vi "ScanningWaveform_v5.vi"(0 "Vy-min":dbl, 1 "Vy-max":dbl, 2 "yPixels/tPixels":dbl, 3 "xPixels/rPixels":dbl, 4 "Vx-min":dbl, 5 "Vx-max":dbl, 6 "Drawing Mode":u16(ring) items=["Image", "Fill Rectangle", "Fill Circle", "Draw Freeform", "Fill Freeform", "Ellipse Boundary", "Line"], 7 "Angle":dbl, 8 "Scanning Mode":u16(ring) items=["Raster", "Spiral"], 9 "AOrate":dbl, 10 "Points":cluster{"X":dbl, "Y":dbl}[](array[cluster]), 11 "points in ellipse":dbl) -> (12 "numPixels":dbl, 13 "Y-WaveArray":dbl[](array[numeric]), 14 "P":dbl, 19 "X-WaveArray":dbl[](array[numeric]))   [LabVIEW 2015]
panel:
  out "Y Graph 2":dbl[](graph)
  out "min":dbl
  out "max":dbl
  out "flyback time (us)":dbl
  out "C":dbl
  out "Sx":dbl
  out "S":dbl
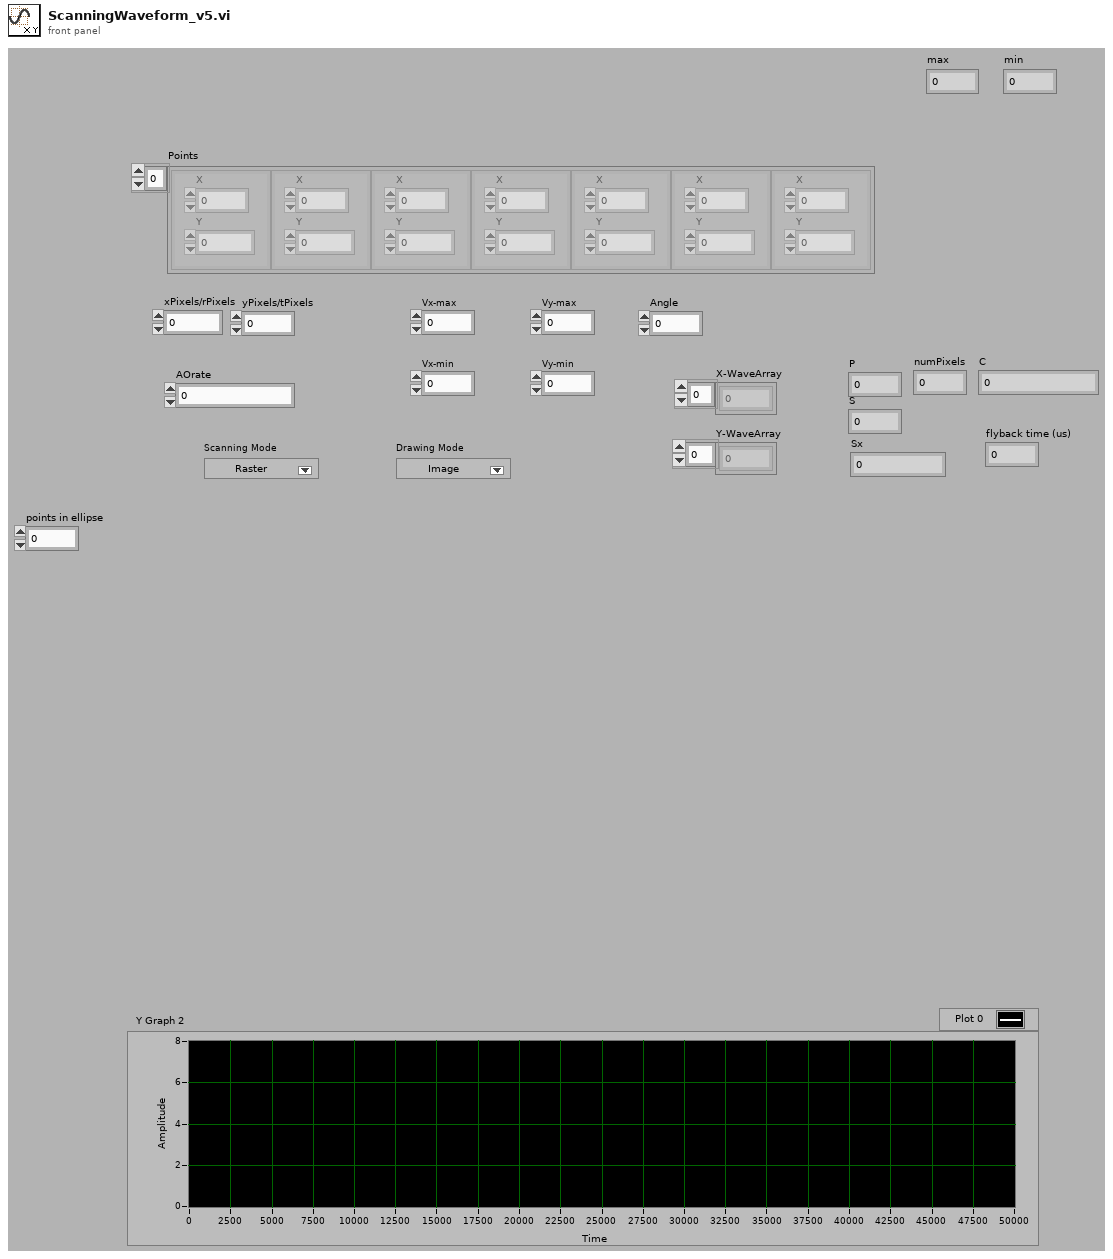
[diagram p1: front panel]
types:
  T1 = typedef "LVRectTypeDef.ctl" = cluster{"Left":i16, "Top":i16, "Right":i16, "Bottom":i16}
  T2 = cluster{"Xpixels":i32, "Vxminref":dbl, "Vxmaxref":dbl, "P":dbl, "Ypixels":i32, "Vyminref":dbl, "Vymaxref":dbl, "srate":sgl, "sAOxy":i32, "timeout":dbl, "type":string, "date":string, "time":string, "Colormap":u16, "Drawing Mode":u16, "Scanning Mode":u16, "square pixels":bool, "square matrix":bool, "Xpixels Img":i32, "Vx-min Img":dbl, "VX-max Img":dbl, "Ypixels Img":i32, "Vy-min Img":dbl, "Vy-max Img ":dbl, "Angle Img":dbl, "autoshutter":bool, "finite":bool, "cont":bool, "wavdet":bool, "measpoints":i32, "avpp":i32, "bufferAO":i32, "bufferAI":i32, "starttick":u32, "waveform":path, "Vx-ref":dbl, "Vy-ref":dbl, "refreshrate":dbl, "refreshbuffer":i32, "tt_cycles":i32, "motorref":refnum<k7>, "mirrorswitch":refnum<k7>, "sample mode":i32, "maxbufferAI":i32, "srateAODO":sgl, "bin":sgl, "Pel":sgl, "Angle draw":dbl, "srate Img":sgl, "ROIimg_plotbounds":T1, "auto OD":bool, "ODfilt":u16, "aAI":i32[], "aCI":i32[], "aAO":u32[], "aDO":u32[], "refwfsize":dbl, "Lifetime":bool, "Vz-Img":dbl, "Vz-ref":dbl, "Vz-reset":dbl, "AIoverride":bool, "aAS":u32[], "XYZstart":dbl[]}
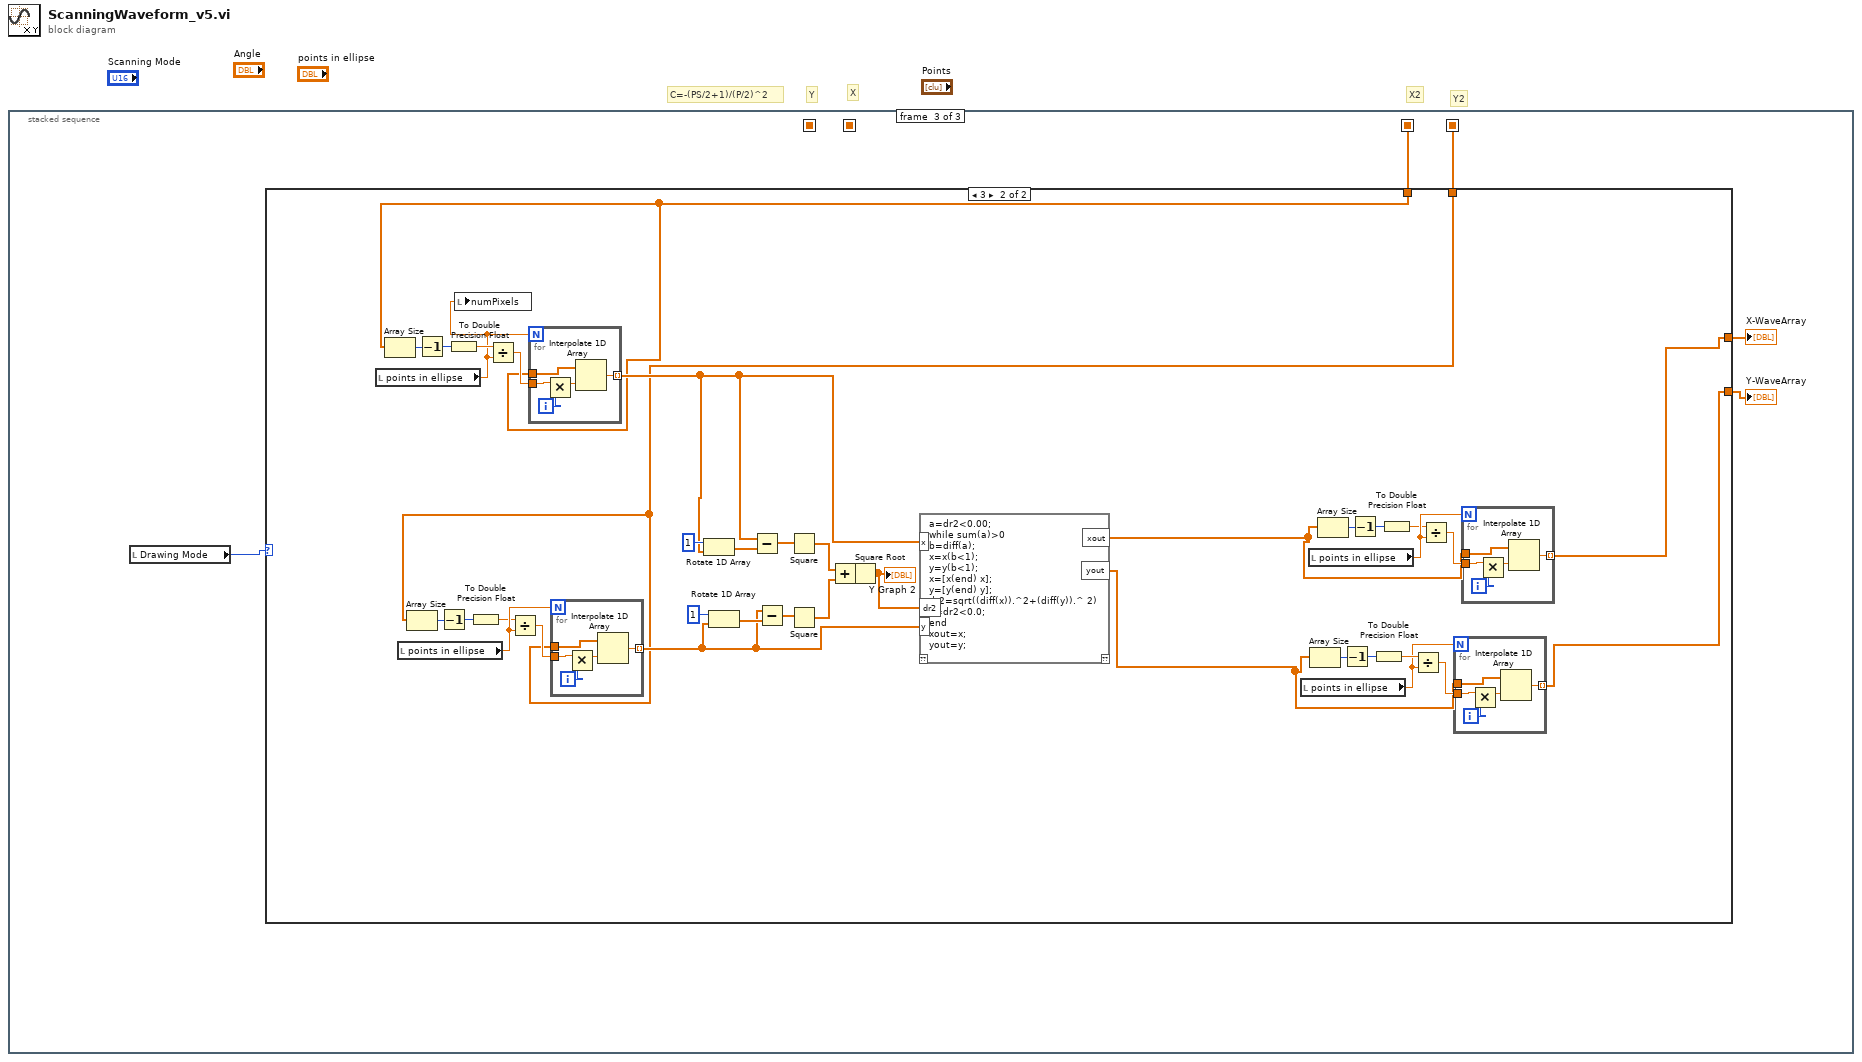
[diagram p0: block diagram]
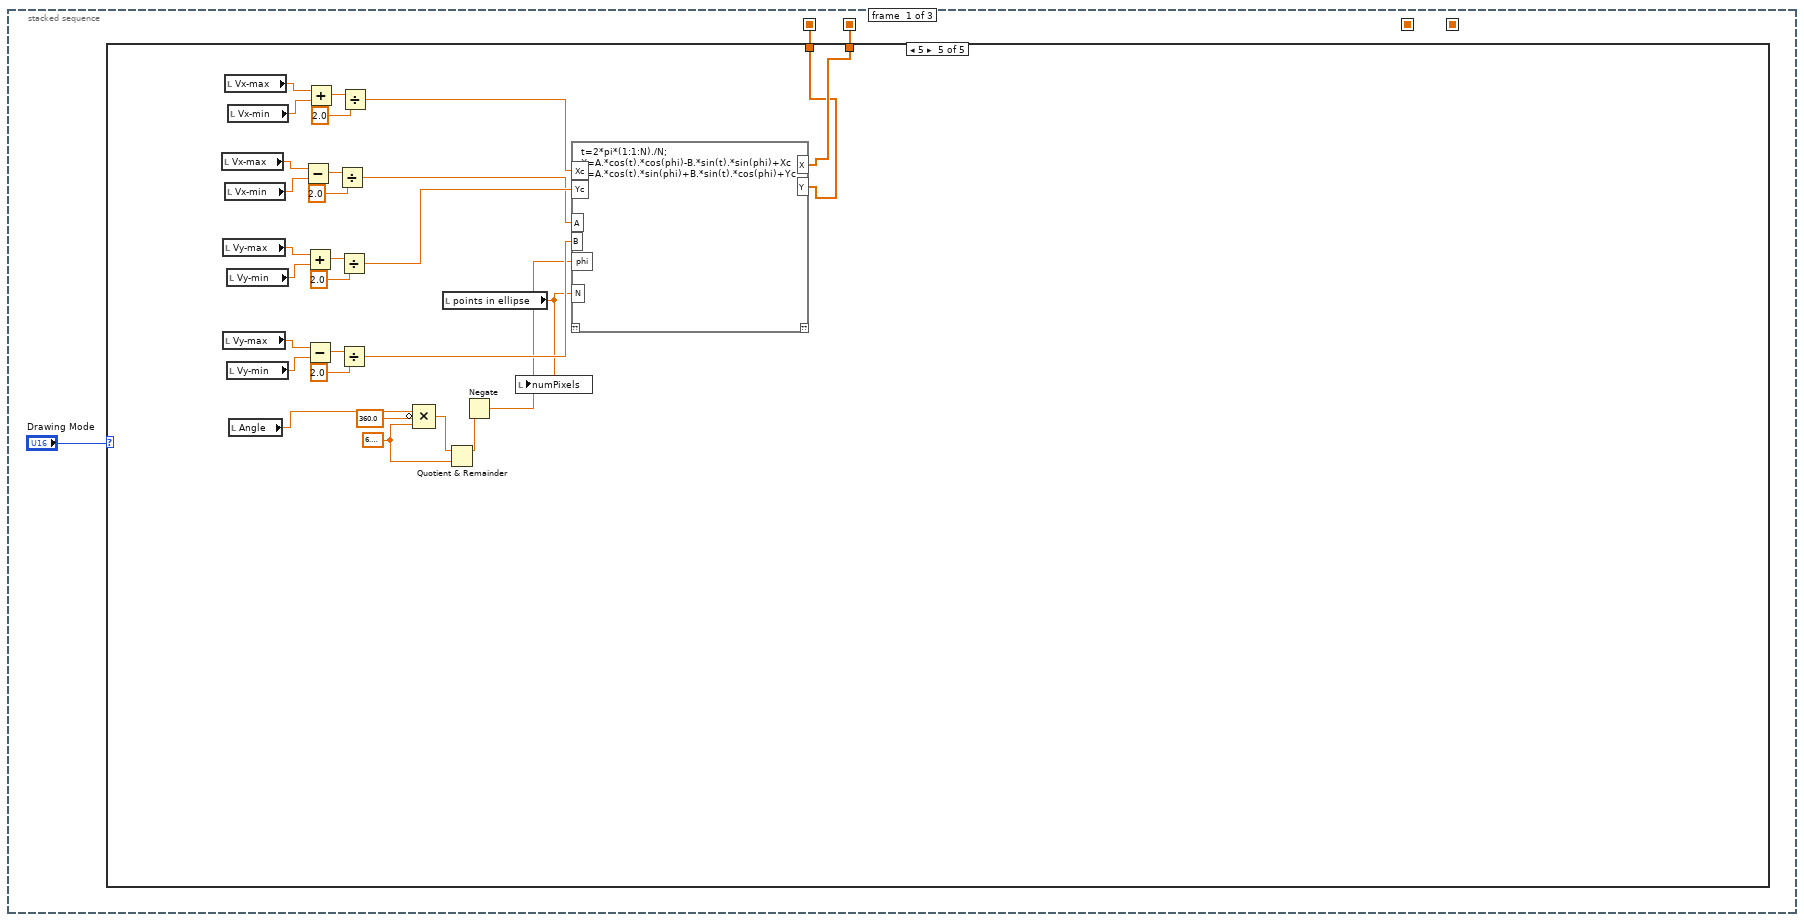
[diagram p2: hidden frame]
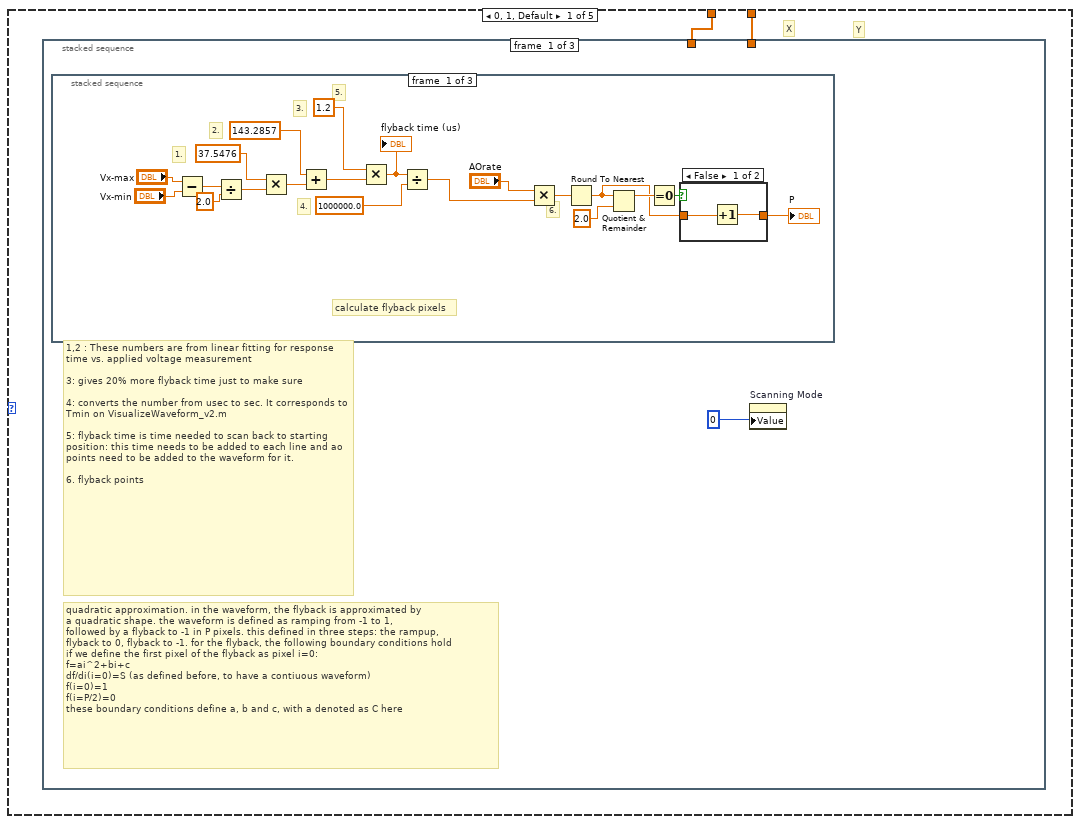
[diagram p3: hidden frame]
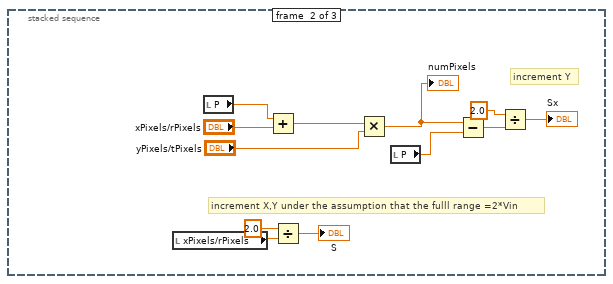
[diagram p5: hidden frame]
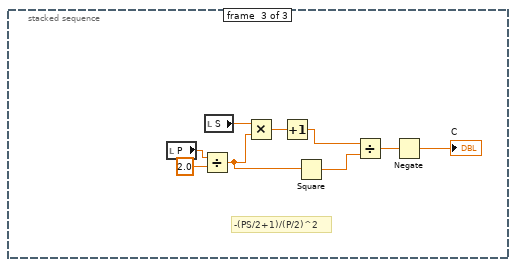
[diagram p6: hidden frame]
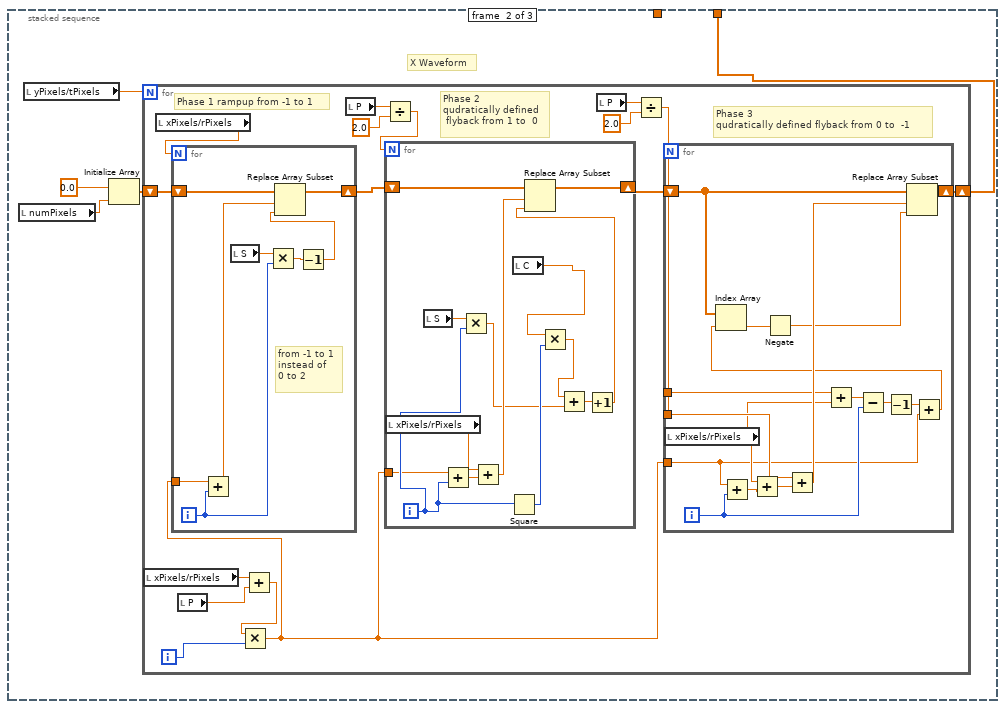
[diagram p7: hidden frame]
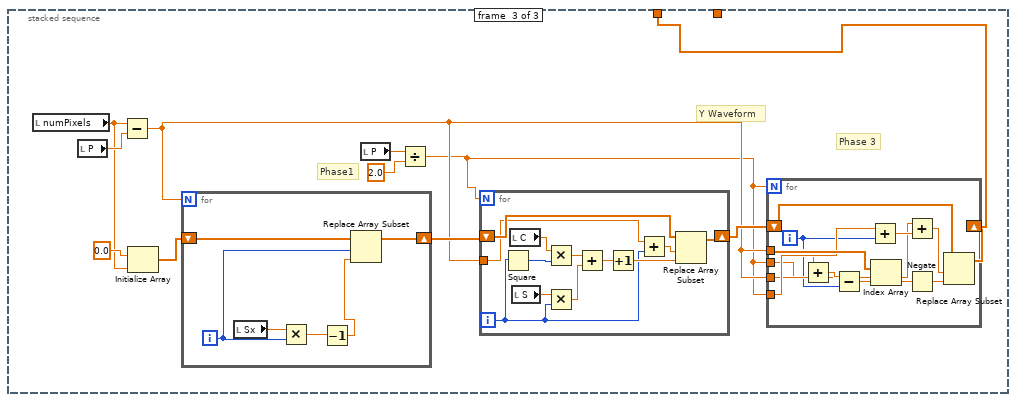
[diagram p8: hidden frame]
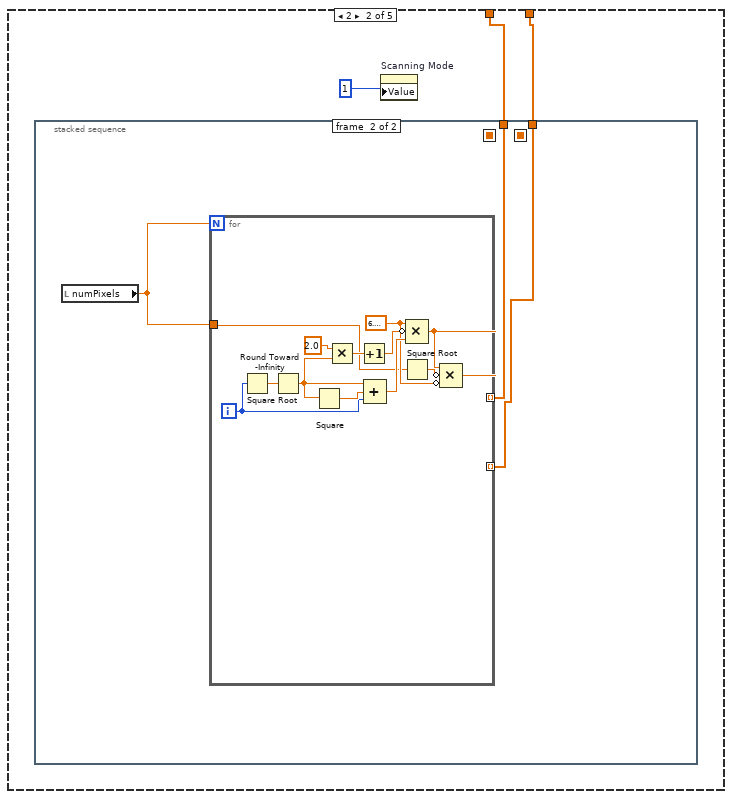
[diagram p9: hidden frame]
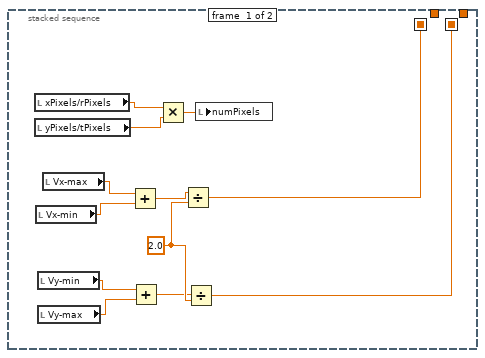
[diagram p10: hidden frame]
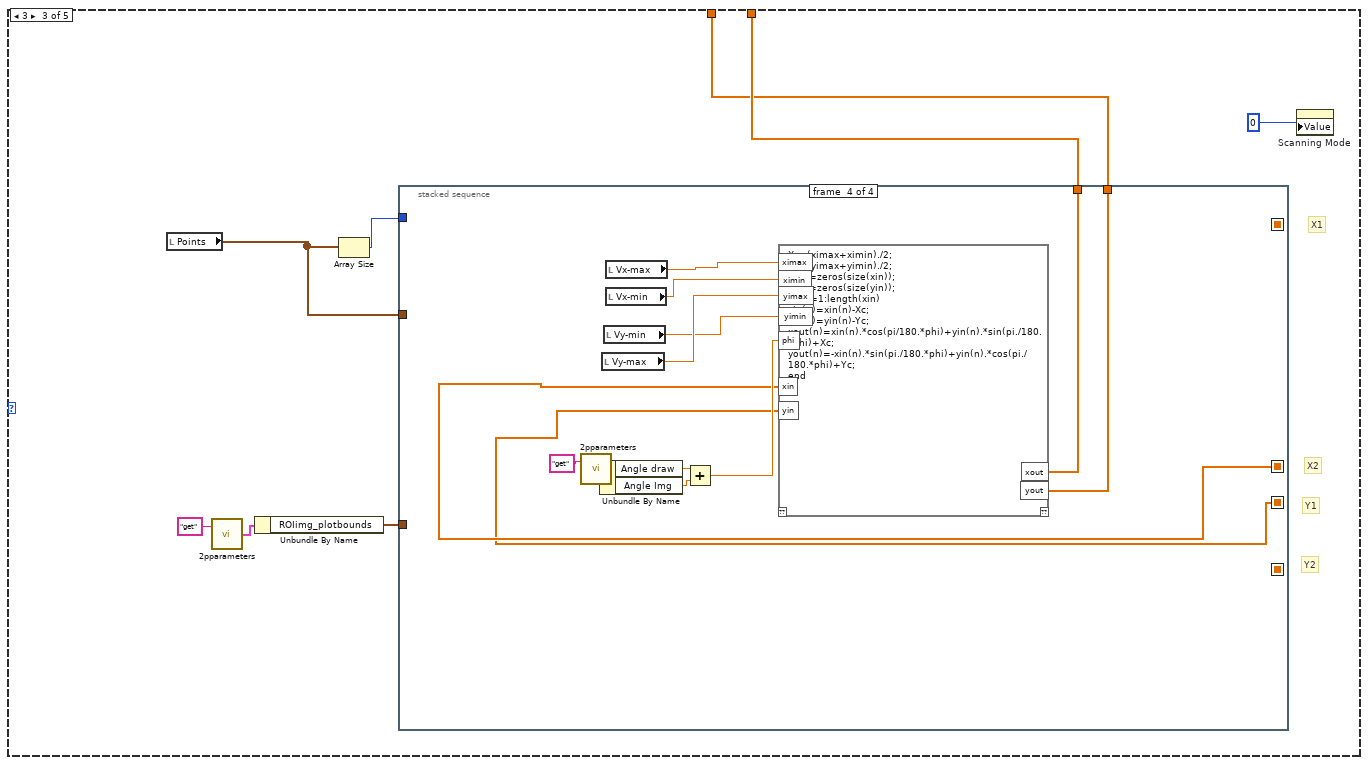
[diagram p11: hidden frame]
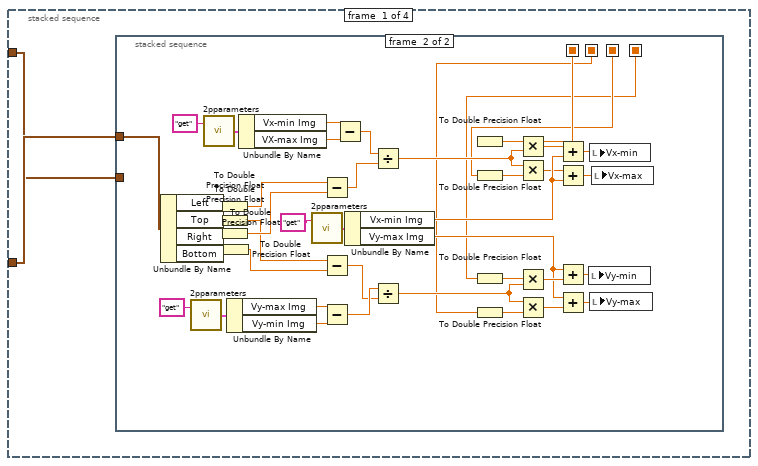
[diagram p12: hidden frame]
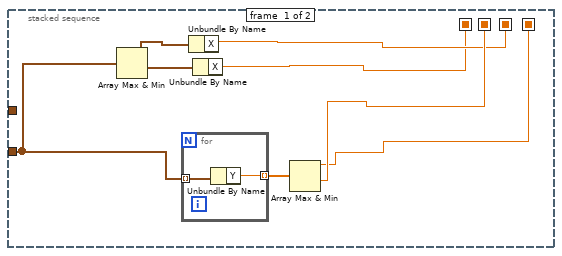
[diagram p13: hidden frame]
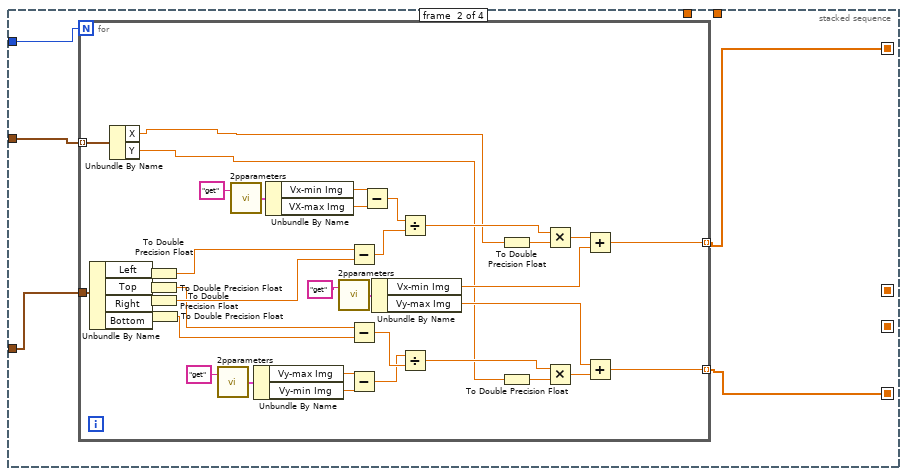
[diagram p14: hidden frame]
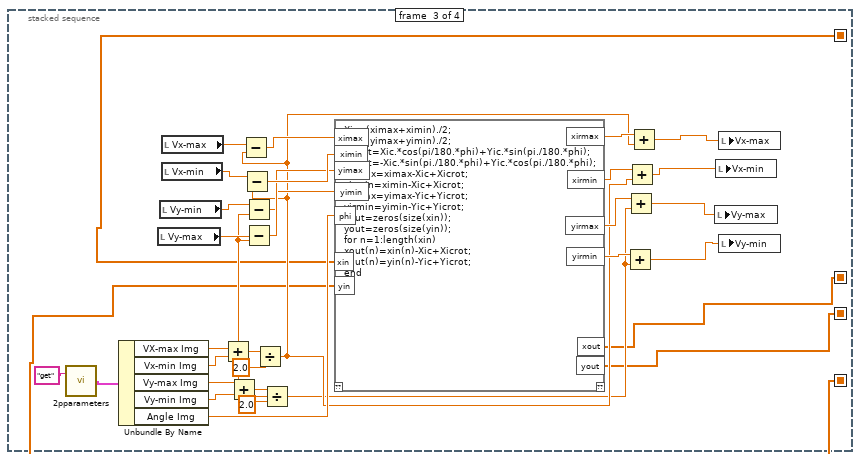
[diagram p15: hidden frame]
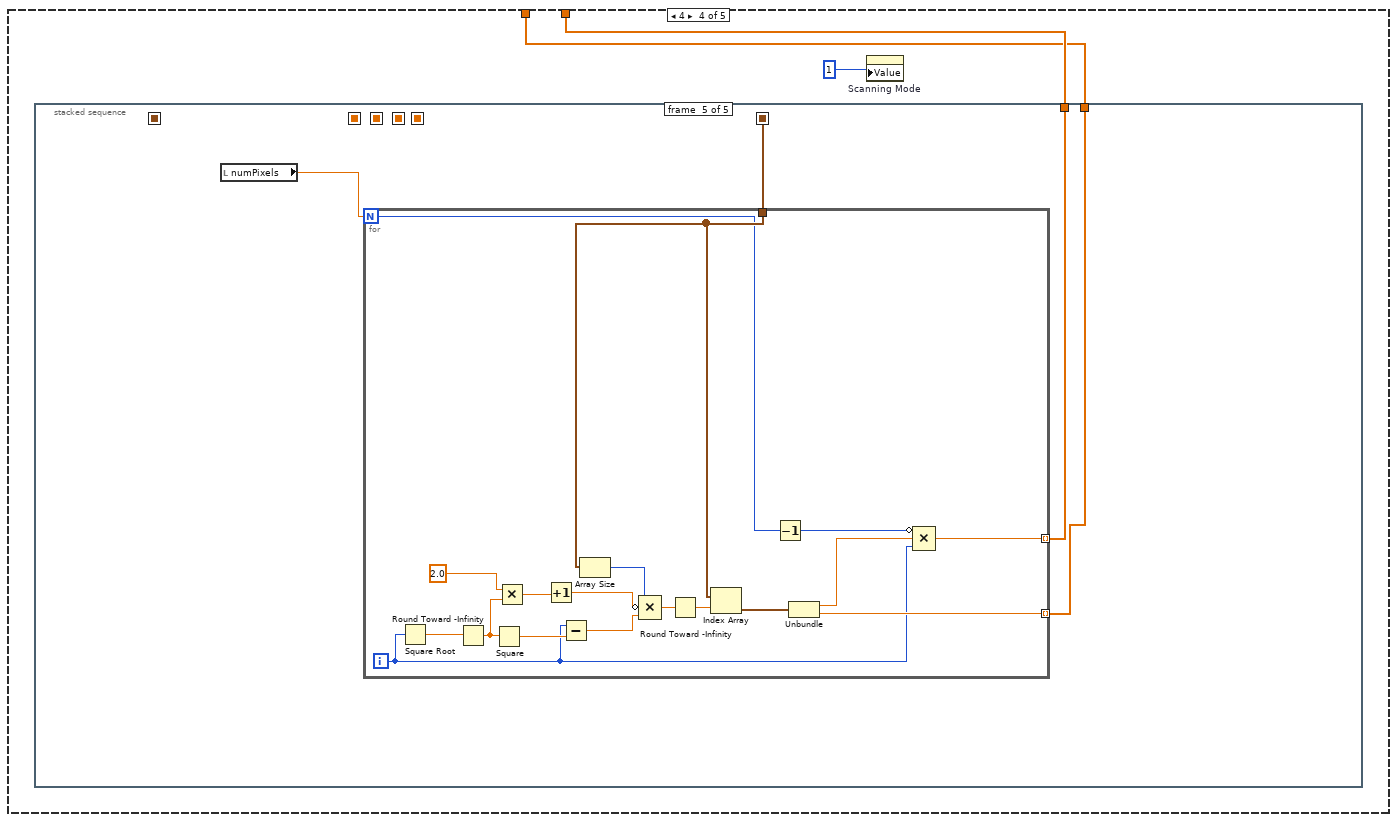
[diagram p16: hidden frame]
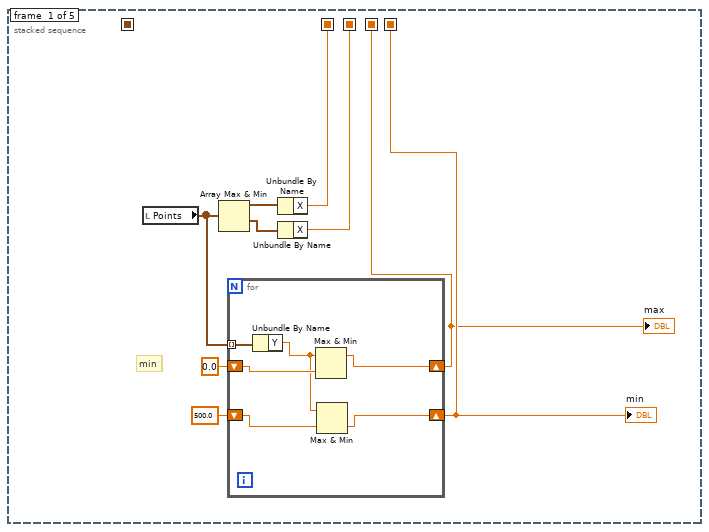
[diagram p17: hidden frame]
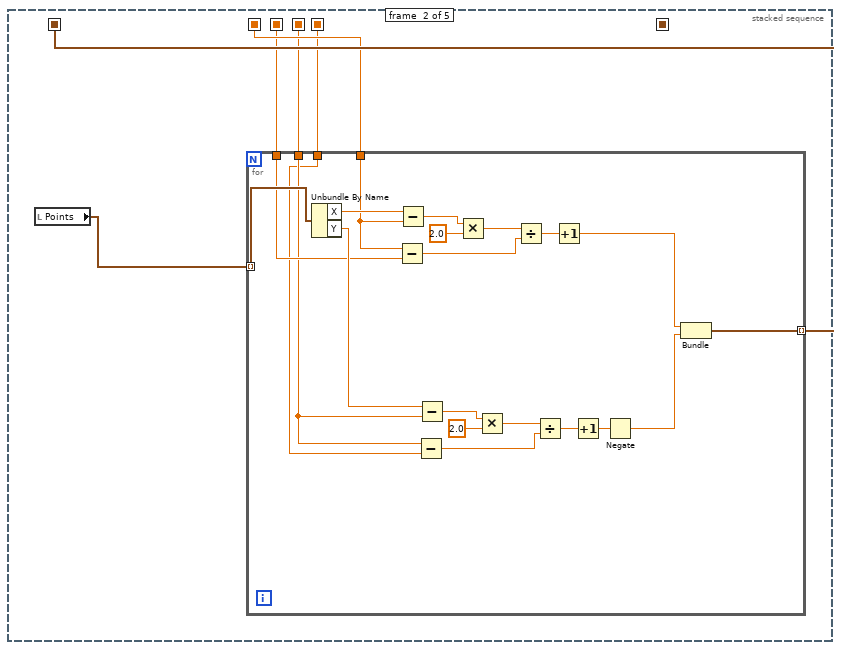
[diagram p18: hidden frame]
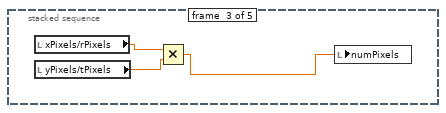
[diagram p19: hidden frame]
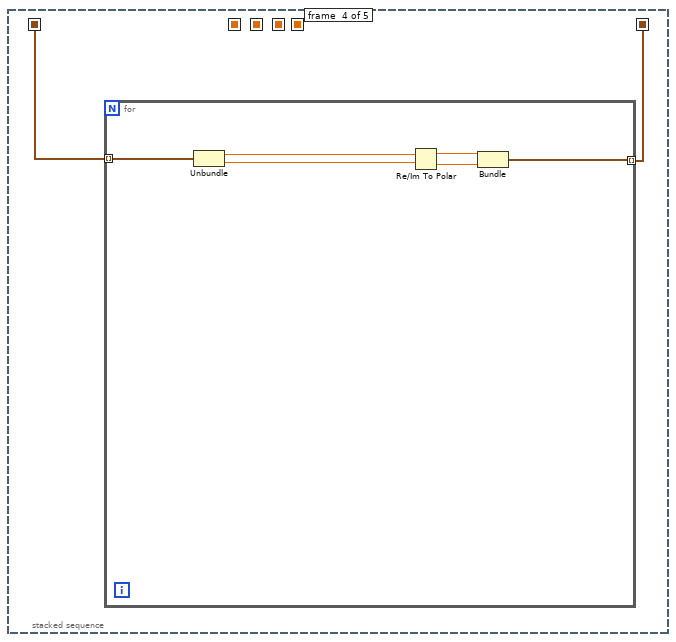
[diagram p20: hidden frame]
diagram:
  # "Y2"
  # "X2"
  # "Y"
  # "X"
  # "C=-(PS/2+1)/(P/2)^2"
  n1 = stacked-sequence {
    seq-local: [w1 _ _] -> [_ w443 _]
    seq-local: [w2 _ _] -> [_ w442 _]
    seq-local: [_ w441 _] -> [_ _ w500]
    seq-local: [_ w440 _] -> [_ _ w497]
    frame #0 {
      n2 = case shown="5" "Drawing Mode" {
        tunnel: [w5 w153 w183 w333 w411] -> w2
        tunnel: [w4 w152 w184 w334 w412] -> w1
        frame 0, 1, Default {
          # "Y"
          # "X"
          n3 = stacked-sequence {
            tunnel: [_ _ w110] -> w5
            tunnel: [_ w51 _] -> w4
            frame #0 {
              # "quadratic approximation. in the waveform, the flyback is approximated by\na quadratic shape. the waveform is defined as ramping from -1 to 1, \nfollowed by a flyback to -1 in P pixels. this defined in three steps: the rampup,\nflyback to 0, flyback to -1. for the flyback, the following boundary conditions hold\nif we define the first pixel of the flyback as pixel i=0:\nf=ai^2+bi+c\ndf/di(i=0)=S (as defined before, to have a contiuous waveform)\nf(i=0)=1\nf(i=P/2)=0\nthese boundary conditions define a, b and c, with a denoted as C here"
              # "1,2 : These numbers are from linear fitting for response time vs. applied voltage measurement\n\n3: gives 20% more flyback time just to make sure\n\n4: converts the number from usec to sec. It corresponds to Tmin on VisualizeWaveform_v2.m\n\n5: flyback time is time needed to scan back to starting position: this time needs to be added to each line and ao points need to be added to the waveform for it.\n\n6. flyback points"
              n4 = stacked-sequence {
                frame #0 {
                  # "calculate flyback pixels"
                  # "6."
                  # "5."
                  # "4."
                  # "3."
                  # "2."
                  # "1."
                  n5 = Subtract(x="Vx-max", y="Vx-min") -> (x-y=w8:dbl)
                  n6 = Divide(x=w8, y=2.0 ("x-y")) -> (x/y=w7:dbl)
                  n7 = Multiply(x=37.5476, y=w7) -> (x*y=w24:dbl)
                  n8 = Add(x=143.2857, y=w24) -> (x+y=w22:dbl)
                  n9 = Multiply(x=1.2, y=w22) -> (x*y=w20:dbl)
                  "flyback time (us)" <- w20
                  n10 = Divide(x=w20, y=1000000.0 ("x")) -> (x/y=w18:dbl)
                  n11 = Multiply(x="AOrate", y=w18) -> (x*y=w17:dbl)
                  n12 = Round To Nearest(number=w17) -> (nearest integer value=w12:dbl)
                  n13 = Quotient & Remainder(x=w12, y=2.0) -> (x-y*floor(x/y)=w14:dbl)  [unwired: 1 out]
                  n14 = Equal To 0?(x=w14) -> (x = 0?=w15:bool)
                  n15 = case shown="False" w15 {
                    tunnel: [w27 w29] -> w13
                    tunnel: w12 -> [w28 w29]
                    frame False {
                      n16 = Increment(x=w28) -> (x+1=w27:dbl)
                    }
                    frame True {
                    }
                  }
                  "P" <- w13
                }
                frame #1 {
                  # "increment X,Y under the assumption that the fulll range =2*Vin"
                  # "increment Y"
                  n17 = local read "xPixels/rPixels"() -> (w34:dbl)
                  n18 = local read "P"() -> (w40:dbl)
                  n19 = Add(x=w40, y="xPixels/rPixels") -> (x+y=w36:dbl)
                  n20 = Divide(x=2.0, y=w34) -> (x/y=→"S":dbl)
                  n21 = Multiply(x=w36, y="yPixels/tPixels") -> (x*y=w39:dbl)
                  "numPixels" <- w39
                  n22 = local read "P"() -> (w41:dbl)
                  n23 = Subtract(x=w39, y=w41) -> (x-y=w32:dbl)
                  n24 = Divide(x=2.0, y=w32) -> (x/y=→"Sx":dbl)
                }
                frame #2 {
                  # "-(PS/2+1)/(P/2)^2"
                  n25 = local read "P"() -> (w48:dbl)
                  n26 = Divide(x=w48, y=2.0) -> (x/y=w50:dbl)
                  n27 = local read "S"() -> (w49:dbl)
                  n28 = Multiply(x=w49, y=w50) -> (x*y=w45:dbl)
                  n29 = Increment(x=w45) -> (x+1=w42:dbl)
                  n30 = Square(x=w50) -> (x^2=w46:dbl)
                  n31 = Divide(x=w42, y=w46) -> (x/y=w47:dbl)
                  n32 = Negate(x=w47) -> (-x=→"C":dbl)
                }
              }
              n33 = property on="Scanning Mode" class="Ring (strict)"("Value"=0) -> ()  [unwired: 2 in, 2 out]
            }
            frame #1 {
              # "X Waveform"
              n34 = local read "numPixels"() -> (w53:dbl)
              n35 = local read "yPixels/tPixels"() -> (w55:dbl)
              n36 = Initialize Array(0.0 ("element"), w53) -> (w52:dbl[])
              n37 = for {
                N: w55 -> [_]
                shift-right: [w57] -> w51
                shift-left: w52 -> [w66]
                i -> [w71]
                # "Phase 3\nqudratically defined flyback from 0 to  -1"
                # "Phase 2\nqudratically defined\n flyback from 1 to  0"
                # "Phase 1 rampup from -1 to 1"
                n38 = local read "xPixels/rPixels"() -> (w70:dbl)
                n39 = local read "xPixels/rPixels"() -> (w67:dbl)
                n40 = local read "P"() -> (w69:dbl)
                n41 = Add(x=w70, y=w69) -> (x+y=w68:dbl)
                n42 = Multiply(x=w68, y=w71) -> (x*y=w56:dbl)
                n43 = for {
                  N: w67 -> [_]
                  shift-right: [w105] -> w58
                  shift-left: w66 -> [w109]
                  tunnel: w56 -> [w104]
                  i -> [w106]
                  # "from -1 to 1\ninstead of\n0 to 2"
                  n44 = Add(x=w104, y=w106) -> (x+y=w108:dbl)
                  n45 = local read "S"() -> (w107:dbl)
                  n46 = Multiply(x=w107, y=w106) -> (x*y=w103:dbl)
                  n47 = Decrement(x=w103) -> (x-1=w102:dbl)
                  n48 = Replace Array Subset(array=w109, new element=w102, index=w108) -> (w105:dbl[])
                }
                n49 = local read "P"() -> (w64:dbl)
                n50 = Divide(x=w64, y=2.0) -> (x/y=w65:dbl)
                n51 = for {
                  N: w65 -> [_]
                  shift-right: [w90] -> w60
                  shift-left: w58 -> [w101]
                  tunnel: w56 -> [w89]
                  i -> [w94]
                  n52 = local read "xPixels/rPixels"() -> (w99:dbl)
                  n53 = local read "S"() -> (w95:dbl)
                  n54 = Add(x=w89, y=w94) -> (x+y=w100:dbl)
                  n55 = Multiply(x=w95, y=w94) -> (x*y=w93:dbl)
                  n56 = Add(x=w99, y=w100) -> (x+y=w98:dbl)
                  n57 = Square(x=w94) -> (x^2=w97:i32)
                  n58 = local read "C"() -> (w88:dbl)
                  n59 = Multiply(x=w88, y=w97) -> (x*y=w96:dbl)
                  n60 = Add(x=w96, y=w93) -> (x+y=w92:dbl)
                  n61 = Increment(x=w92) -> (x+1=w91:dbl)
                  n62 = Replace Array Subset(array=w101, new element=w91, index=w98) -> (w90:dbl[])
                }
                n63 = local read "P"() -> (w61:dbl)
                n64 = Divide(x=w61, y=2.0) -> (x/y=w59:dbl)
                n65 = for {
                  N: w59 -> [_]
                  tunnel: w59 -> [w85]
                  tunnel: w59 -> [w82]
                  shift-right: [w73] -> w57
                  shift-left: w60 -> [w83]
                  tunnel: w56 -> [w72]
                  i -> [w79]
                  n66 = local read "xPixels/rPixels"() -> (w81:dbl)
                  n67 = Add(x=w72, y=w79) -> (x+y=w87:dbl)
                  n68 = Add(x=w81, y=w87) -> (x+y=w86:dbl)
                  n69 = Add(x=w85, y=w86) -> (x+y=w84:dbl)
                  n70 = Add(x=w82, y=w81) -> (x+y=w80:dbl)
                  n71 = Subtract(x=w80, y=w79) -> (x-y=w78:dbl)
                  n72 = Decrement(x=w78) -> (x-1=w77:dbl)
                  n73 = Add(x=w77, y=w72) -> (x+y=w76:dbl)
                  n74 = Index Array(array=w83, index=w76) -> (element=w75:dbl)
                  n75 = Negate(x=w75) -> (-x=w74:dbl)
                  n76 = Replace Array Subset(array=w83, new element=w74, index=w84) -> (w73:dbl[])
                }
              }
            }
            frame #2 {
              # "Phase 3"
              # "Phase1"
              # "Y Waveform"
              n77 = local read "numPixels"() -> (w117:dbl)
              n78 = local read "P"() -> (w118:dbl)
              n79 = Subtract(x=w117, y=w118) -> (x-y=w112:dbl)
              n80 = Initialize Array(0.0 ("element"), w117) -> (w119:dbl[])
              n81 = for {
                N: w112 -> [_]
                shift-right: [w148] -> w114
                shift-left: w119 -> [w151]
                i -> [w149]
                n82 = local read "Sx"() -> (w150:dbl)
                n83 = Multiply(x=w150, y=w149) -> (x*y=w146:dbl)
                n84 = Decrement(x=w146) -> (x-1=w147:dbl)
                n85 = Replace Array Subset(array=w151, new element=w147, index=w149) -> (w148:dbl[])
              }
              n86 = local read "P"() -> (w116:dbl)
              n87 = Divide(x=w116, y=2.0) -> (x/y=w111:dbl)
              n88 = for {
                N: w111 -> [_]
                shift-right: [w138] -> w113
                shift-left: w114 -> [w145]
                tunnel: w112 -> [w137]
                i -> [w135]
                n89 = Square(x=w135) -> (x^2=w143:i32)
                n90 = local read "C"() -> (w134:dbl)
                n91 = local read "S"() -> (w136:dbl)
                n92 = Multiply(x=w134, y=w143) -> (x*y=w142:dbl)
                n93 = Multiply(x=w136, y=w135) -> (x*y=w141:dbl)
                n94 = Add(x=w142, y=w141) -> (x+y=w140:dbl)
                n95 = Increment(x=w140) -> (x+1=w139:dbl)
                n96 = Add(x=w137, y=w135) -> (x+y=w144:dbl)
                n97 = Replace Array Subset(array=w145, new element=w139, index=w144) -> (w138:dbl[])
              }
              n98 = for {
                N: w111 -> [_]
                shift-right: [w127] -> w110
                shift-left: w113 -> [w131]
                tunnel: w111 -> [w126]
                tunnel: w112 -> [w125]
                tunnel: w112 -> [w124]
                tunnel: w111 -> [w123]
                i -> [w121]
                n99 = Add(x=w124, y=w123) -> (x+y=w130:dbl)
                n100 = Subtract(x=w130, y=w121) -> (x-y=w122:dbl)
                n101 = Add(x=w126, y=w121) -> (x+y=w133:dbl)
                n102 = Index Array(array=w131, index=w122) -> (element=w129:dbl)
                n103 = Add(x=w125, y=w133) -> (x+y=w132:dbl)
                n104 = Negate(x=w129) -> (-x=w128:dbl)
                n105 = Replace Array Subset(array=w131, new element=w128, index=w132) -> (w127:dbl[])
              }
            }
          }
        }
        frame 2 {
          n106 = stacked-sequence {
            seq-local: [w156 _] -> [_ _]
            seq-local: [w160 _] -> [_ _]
            tunnel: [_ w168] -> w153
            tunnel: [_ w167] -> w152
            frame #0 {
              w164 = 2.0
              n107 = local read "xPixels/rPixels"() -> (w166:dbl)
              n108 = local read "yPixels/tPixels"() -> (w165:dbl)
              n109 = local read "Vx-min"() -> (w162:dbl)
              n110 = local read "Vy-min"() -> (w159:dbl)
              n111 = local read "Vy-max"() -> (w158:dbl)
              n112 = local read "Vx-max"() -> (w163:dbl)
              n113 = Add(x=w163, y=w162) -> (x+y=w161:dbl)
              n114 = Add(x=w159, y=w158) -> (x+y=w157:dbl)
              n115 = Multiply(x=w166, y=w165) -> (x*y=w155:dbl)
              n116 = Divide(x=w161, y=w164) -> (x/y=w160:dbl)
              n117 = Divide(x=w157, y=w164) -> (x/y=w156:dbl)
              n118 = local write "numPixels"(w155) -> ()
            }
            frame #1 {
              n119 = local read "numPixels"() -> (w169:dbl)
              n120 = for {
                N: w169 -> [_]
                tunnel: w169 -> [w171]
                tunnel: [w176] -> w167 mode=indexing
                tunnel: [w177] -> w168 mode=indexing
                i -> [w174]
                w172 = 6.283185307179586
                n121 = Square Root(x=w174) -> (sqrt(x)=w182:dbl)
                n122 = Round Toward -Infinity(1:w182) -> (0:w173:dbl)
                n123 = Square(x=w173) -> (x^2=w181:dbl)
                n124 = Multiply(x=2.0, y=w173) -> (x*y=w180:dbl)
                n125 = Increment(x=w180) -> (x+1=w179:dbl)
                n126 = Compound Arithmetic op=ADD(w173, w181, w174) -> (w175:dbl)
                n127 = Square Root(x=w171) -> (sqrt(x)=w170:dbl)
                n128 = Compound Arithmetic op=MULTIPLY(w172, invert w179, w175) -> (w177:dbl)
                n129 = Compound Arithmetic op=MULTIPLY(w177, invert w170, invert w172) -> (w176:dbl)
              }
            }
          }
          n130 = property on="Scanning Mode" class="Ring (strict)"("Value"=1) -> ()  [unwired: 2 in, 2 out]
        }
        frame 3 {
          # "Y2"
          # "X1"
          # "Y1"
          # "X2"
          n131 = local read "Points"() -> (w187:cluster{"X":dbl, "Y":dbl}[])
          n132 = call "2pparameters.vi"("command"="get") -> ("params out"=w185:T2)  [unwired: 1 in]
          n133 = Unbundle By Name(w185) -> ("ROIimg_plotbounds"=w186:T1)
          n134 = Array Size(array=w187) -> (size(s)=w188:i32)
          n135 = stacked-sequence {
            seq-local: [_ w246 _ _] -> [_ _ w290 _]
            seq-local: [_ w247 _ _] -> [_ _ w289 _]
            seq-local: [_ _ w288 _] -> [_ _ _ w323]
            seq-local: [_ _ w287 _] -> [_ _ _ w322]
            tunnel: w187 -> [w191 w249 _ _]
            tunnel: w186 -> [w192 w250 _ _]
            tunnel: w188 -> [_ w248 _ _]
            tunnel: [_ _ _ w321] -> w184
            tunnel: [_ _ _ w320] -> w183
            frame #0 {
              n136 = stacked-sequence {
                seq-local: [w193 _] -> [_ w207]
                seq-local: [w196 _] -> [_ w206]
                seq-local: [w194 _] -> [_ w205]
                seq-local: [w195 _] -> [_ w204]
                tunnel: w191 -> [w200 _]
                tunnel: w192 -> [_ w203]
                frame #0 {
                  n137 = Array Max & Min(array=w200) -> (max value=w199:cluster{"X":dbl, "Y":dbl}, min value=w198:cluster{"X":dbl, "Y":dbl})  [unwired: 2 out]
                  n138 = for {
                    tunnel: w200 -> [w202] mode=indexing
                    tunnel: [w201] -> w197 mode=indexing
                    n139 = Unbundle By Name(w202) -> ("Y"=w201:dbl)
                  }
                  n140 = Unbundle By Name(w199) -> ("X"=w194:dbl)
                  n141 = Unbundle By Name(w198) -> ("X"=w193:dbl)
                  n142 = Array Max & Min(array=w197) -> (max value=w195:dbl, min value=w196:dbl)  [unwired: 2 out]
                }
                frame #1 {
                  n143 = Unbundle By Name(w203) -> ("Left"=w208:i16, "Top"=w209:i16, "Right"=w210:i16, "Bottom"=w211:i16)
                  n144 = call "2pparameters.vi"("command"="get") -> ("params out"=w229:T2)  [unwired: 1 in]
                  n145 = call "2pparameters.vi"("command"="get") -> ("params out"=w217:T2)  [unwired: 1 in]
                  n146 = To Double Precision Float(number=w208) -> (double precision float=w244:dbl)
                  n147 = To Double Precision Float(number=w209) -> (double precision float=w212:dbl)
                  n148 = To Double Precision Float(number=w210) -> (double precision float=w245:dbl)
                  n149 = To Double Precision Float(number=w211) -> (double precision float=w213:dbl)
                  n150 = Unbundle By Name(w229) -> ("Vy-max Img"=w231:dbl, "Vy-min Img"=w232:dbl)
                  n151 = Unbundle By Name(w217) -> ("Vx-min Img"=w223:dbl, "VX-max Img"=w218:dbl)
                  n152 = call "2pparameters.vi"("command"="get") -> ("params out"=w222:T2)  [unwired: 1 in]
                  n153 = Subtract(x=w244, y=w245) -> (x-y=w214:dbl)
                  n154 = Subtract(x=w212, y=w213) -> (x-y=w215:dbl)
                  n155 = Subtract(x=w231, y=w232) -> (x-y=w233:dbl)
                  n156 = Subtract(x=w223, y=w218) -> (x-y=w219:dbl)
                  n157 = Unbundle By Name(w222) -> ("Vx-min Img"=w227:dbl, "Vy-max Img"=w235:dbl)
                  n158 = Divide(x=w219, y=w214) -> (x/y=w241:dbl)
                  n159 = Divide(x=w233, y=w215) -> (x/y=w242:dbl)
                  n160 = To Double Precision Float(number=w207) -> (double precision float=w240:dbl)
                  n161 = To Double Precision Float(number=w205) -> (double precision float=w225:dbl)
                  n162 = To Double Precision Float(number=w204) -> (double precision float=w234:dbl)
                  n163 = To Double Precision Float(number=w206) -> (double precision float=w243:dbl)
                  n164 = Multiply(x=w240, y=w241) -> (x*y=w224:dbl)
                  n165 = Multiply(x=w241, y=w225) -> (x*y=w226:dbl)
                  n166 = Multiply(x=w234, y=w242) -> (x*y=w236:dbl)
                  n167 = Multiply(x=w242, y=w243) -> (x*y=w237:dbl)
                  n168 = Add(x=w224, y=w227) -> (x+y=w220:dbl)
                  n169 = Add(x=w226, y=w227) -> (x+y=w228:dbl)
                  n170 = Add(x=w235, y=w236) -> (x+y=w238:dbl)
                  n171 = Add(x=w235, y=w237) -> (x+y=w239:dbl)
                  n172 = local write "Vy-min"(w238) -> ()
                  n173 = local write "Vx-min"(w220) -> ()
                  n174 = local write "Vy-max"(w239) -> ()
                  n175 = local write "Vx-max"(w228) -> ()
                }
              }
            }
            frame #1 {
              n176 = for {
                N: w248 -> [_]
                tunnel: w250 -> [w258]
                tunnel: w249 -> [w257] mode=indexing
                tunnel: [w254] -> w246 mode=indexing
                tunnel: [w253] -> w247 mode=indexing
                n177 = Unbundle By Name(w258) -> ("Left"=w286:i16, "Top"=w285:i16, "Right"=w284:i16, "Bottom"=w283:i16)
                n178 = Unbundle By Name(w257) -> ("X"=w252:dbl, "Y"=w251:dbl)
                n179 = To Double Precision Float(number=w286) -> (double precision float=w256:dbl)
                n180 = To Double Precision Float(number=w285) -> (double precision float=w255:dbl)
                n181 = To Double Precision Float(number=w284) -> (double precision float=w259:dbl)
                n182 = To Double Precision Float(number=w283) -> (double precision float=w282:dbl)
                n183 = call "2pparameters.vi"("command"="get") -> ("params out"=w269:T2)  [unwired: 1 in]
                n184 = call "2pparameters.vi"("command"="get") -> ("params out"=w278:T2)  [unwired: 1 in]
                n185 = Unbundle By Name(w269) -> ("Vy-max Img"=w267:dbl, "Vy-min Img"=w266:dbl)
                n186 = Unbundle By Name(w278) -> ("Vx-min Img"=w273:dbl, "VX-max Img"=w277:dbl)
                n187 = call "2pparameters.vi"("command"="get") -> ("params out"=w274:T2)  [unwired: 1 in]
                n188 = Subtract(x=w256, y=w259) -> (x-y=w281:dbl)
                n189 = Subtract(x=w255, y=w282) -> (x-y=w280:dbl)
                n190 = Subtract(x=w267, y=w266) -> (x-y=w265:dbl)
                n191 = Subtract(x=w273, y=w277) -> (x-y=w276:dbl)
                n192 = Unbundle By Name(w274) -> ("Vx-min Img"=w270:dbl, "Vy-max Img"=w264:dbl)
                n193 = Divide(x=w276, y=w281) -> (x/y=w262:dbl)
                n194 = Divide(x=w265, y=w280) -> (x/y=w261:dbl)
                n195 = To Double Precision Float(number=w252) -> (double precision float=w272:dbl)
                n196 = To Double Precision Float(number=w251) -> (double precision float=w260:dbl)
                n197 = Multiply(x=w262, y=w272) -> (x*y=w271:dbl)
                n198 = Multiply(x=w261, y=w260) -> (x*y=w263:dbl)
                n199 = Add(x=w271, y=w270) -> (x+y=w254:dbl)
                n200 = Add(x=w264, y=w263) -> (x+y=w253:dbl)
              }
            }
            frame #2 {
              n201 = call "2pparameters.vi"("command"="get") -> ("params out"=w302:T2)  [unwired: 1 in]
              n202 = Unbundle By Name(w302) -> ("VX-max Img"=w304:dbl, "Vx-min Img"=w305:dbl, "Vy-max Img"=w306:dbl, "Vy-min Img"=w307:dbl, "Angle Img"=w297:dbl)
              n203 = local read "Vy-max"() -> (w314:dbl)
              n204 = local read "Vy-min"() -> (w315:dbl)
              n205 = local read "Vx-max"() -> (w312:dbl)
              n206 = local read "Vx-min"() -> (w313:dbl)
              n207 = Add(x=w304, y=w305) -> (x+y=w308:dbl)
              n208 = Add(x=w306, y=w307) -> (x+y=w311:dbl)
              n209 = Divide(x=w308, y=2.0) -> (x/y=w292:dbl)
              n210 = Subtract(x=w312, y=w292) -> (x-y=w301:dbl)
              n211 = Subtract(x=w313, y=w292) -> (x-y=w300:dbl)
              n212 = Divide(x=w311, y=2.0) -> (x/y=w291:dbl)
              n213 = Subtract(x=w315, y=w291) -> (x-y=w298:dbl)
              n214 = Subtract(x=w314, y=w291) -> (x-y=w299:dbl)
              n215 = script code="Xic=(ximax+ximin)./2;\nYic=(yimax+yimin)./2;\nXicrot=Xic.*cos(pi/180.*phi)+Yic.*sin(pi./180.*phi);\nYicrot=-Xic.*sin(pi./180.*phi)+Yic.*cos(pi./180.*phi);\nxirmax=ximax-Xic+Xicrot;\nxirmin=ximin-Xic+Xicrot;\nyirmax=yimax-Yic+Yicrot;\nyirmin=yimin-Yic+Yicrot;\nxout=zeros(size(xin));\nyout=zeros(size(yin));\nfor n=1:length(xin)\nxout(n)=xin(n)-Xic+Xicrot;\nyout(n)=yin(n)-Yic+Yicrot;\nend"("ximax"=w301, "ximin"=w300, "yimax"=w299, "yimin"=w298, "phi"=w297, "xin"=w290, "yin"=w289) -> ("xirmax"=w296:dbl, "xirmin"=w295:dbl, "yirmax"=w294:dbl, "yirmin"=w293:dbl, "xout"=w288:dbl[], "yout"=w287:dbl[])  [unwired: 1 in, 1 out]
              n216 = Add(x=w293, y=w291) -> (x+y=w319:dbl)
              n217 = Add(x=w294, y=w291) -> (x+y=w318:dbl)
              n218 = Add(x=w295, y=w292) -> (x+y=w317:dbl)
              n219 = Add(x=w296, y=w292) -> (x+y=w316:dbl)
              n220 = local write "Vy-max"(w318) -> ()
              n221 = local write "Vx-min"(w317) -> ()
              n222 = local write "Vx-max"(w316) -> ()
              n223 = local write "Vy-min"(w319) -> ()
            }
            frame #3 {
              n224 = call "2pparameters.vi"("command"="get") -> ("params out"=w329:T2)  [unwired: 1 in]
              n225 = Unbundle By Name(w329) -> ("Angle draw"=w330:dbl, "Angle Img"=w331:dbl)
              n226 = local read "Vy-max"() -> (w327:dbl)
              n227 = local read "Vy-min"() -> (w326:dbl)
              n228 = local read "Vx-max"() -> (w324:dbl)
              n229 = local read "Vx-min"() -> (w325:dbl)
              n230 = Add(x=w330, y=w331) -> (x+y=w332:dbl)
              n231 = script code="Xc=(ximax+ximin)./2;\nYc=(yimax+yimin)./2;\nxout=zeros(size(xin));\nyout=zeros(size(yin));\nfor n=1:length(xin)\nxin(n)=xin(n)-Xc;\nyin(n)=yin(n)-Yc;\nxout(n)=xin(n).*cos(pi/180.*phi)+yin(n).*sin(pi./180.*phi)+Xc;\nyout(n)=-xin(n).*sin(pi./180.*phi)+yin(n).*cos(pi./180.*phi)+Yc;\nend"("ximax"=w324, "ximin"=w325, "yimax"=w327, "yimin"=w326, "phi"=w332, "xin"=w323, "yin"=w322) -> ("xout"=w321:dbl[], "yout"=w320:dbl[])  [unwired: 1 in, 1 out]
            }
          }
          n232 = property on="Scanning Mode" class="Ring (strict)"("Value"=0) -> ()  [unwired: 2 in, 2 out]
        }
        frame 4 {
          n233 = stacked-sequence {
            seq-local: [_ _ _ w381 _] -> [_ _ _ _ w391]
            seq-local: [_ w355 _ _ _] -> [_ _ _ w382 _]
            seq-local: [w341 _ _ _ _] -> [_ w354 _ _ _]
            seq-local: [w340 _ _ _ _] -> [_ w353 _ _ _]
            seq-local: [w338 _ _ _ _] -> [_ w352 _ _ _]
            seq-local: [w339 _ _ _ _] -> [_ w351 _ _ _]
            tunnel: [_ _ _ _ w390] -> w334
            tunnel: [_ _ _ _ w389] -> w333
            frame #0 {
              # "min"
              # "max"
              n234 = local read "Points"() -> (w342:cluster{"X":dbl, "Y":dbl}[])
              n235 = Array Max & Min(array=w342) -> (max value=w344:cluster{"X":dbl, "Y":dbl}, min value=w343:cluster{"X":dbl, "Y":dbl})  [unwired: 2 out]
              n236 = for {
                tunnel: w342 -> [w350] mode=indexing
                shift-right: [w346] -> w338
                shift-left: 0.0 -> [w349]
                shift-right: [w345] -> w339
                shift-left: 500.0 -> [w347]
                n237 = Unbundle By Name(w350) -> ("Y"=w348:dbl)
                n238 = Max & Min(x=w348, y=w349) -> (max(x,y)=w346:dbl)  [unwired: 1 out]
                n239 = Max & Min(x=w348, y=w347) -> (min(x,y)=w345:dbl)  [unwired: 1 out]
              }
              "max" <- w338
              "min" <- w339
              n240 = Unbundle By Name(w344) -> ("X"=w341:dbl)
              n241 = Unbundle By Name(w343) -> ("X"=w340:dbl)
            }
            frame #1 {
              n242 = local read "Points"() -> (w356:cluster{"X":dbl, "Y":dbl}[])
              n243 = for {
                tunnel: w356 -> [w377] mode=indexing
                tunnel: [w376] -> w355 mode=indexing
                tunnel: w354 -> [w362]
                tunnel: w353 -> [w361]
                tunnel: w352 -> [w360]
                tunnel: w351 -> [w359]
                n244 = Unbundle By Name(w377) -> ("X"=w364:dbl, "Y"=w363:dbl)
                n245 = Subtract(x=w362, y=w361) -> (x-y=w371:dbl)
                n246 = Subtract(x=w364, y=w362) -> (x-y=w372:dbl)
                n247 = Subtract(x=w360, y=w359) -> (x-y=w366:dbl)
                n248 = Subtract(x=w363, y=w360) -> (x-y=w367:dbl)
                n249 = Multiply(x=w372, y=2.0) -> (x*y=w373:dbl)
                n250 = Multiply(x=w367, y=2.0) -> (x*y=w368:dbl)
                n251 = Divide(x=w373, y=w371) -> (x/y=w375:dbl)
                n252 = Divide(x=w368, y=w366) -> (x/y=w369:dbl)
                n253 = Increment(x=w375) -> (x+1=w374:dbl)
                n254 = Increment(x=w369) -> (x+1=w358:dbl)
                n255 = Negate(x=w358) -> (-x=w357:dbl)
                n256 = Bundle(w374, w357) -> (w376:cluster{dbl, dbl})  [unwired: 1 in]
              }
            }
            frame #2 {
              n257 = local read "xPixels/rPixels"() -> (w380:dbl)
              n258 = local read "yPixels/tPixels"() -> (w379:dbl)
              n259 = Multiply(x=w380, y=w379) -> (x*y=w378:dbl)
              n260 = local write "numPixels"(w378) -> ()
            }
            frame #3 {
              n261 = for {
                tunnel: w382 -> [w388] mode=indexing
                tunnel: [w385] -> w381 mode=indexing
                n262 = Unbundle(w388) -> (w387:dbl, w386:dbl)
                n263 = Re/Im To Polar(2:w386, 3:w387) -> (0:w383:dbl, 1:w384:dbl)
                n264 = Bundle(w384, w383) -> (w385:cluster{dbl, dbl})  [unwired: 1 in]
              }
            }
            frame #4 {
              n265 = local read "numPixels"() -> (w392:dbl)
              n266 = for {
                N: w392 -> [w394]
                tunnel: w391 -> [w401]
                tunnel: [w399] -> w389 mode=indexing
                tunnel: [w398] -> w390 mode=indexing
                i -> [w396]
                n267 = Square Root(x=w396) -> (sqrt(x)=w409:dbl)
                n268 = Round Toward -Infinity(1:w409) -> (0:w407:dbl)
                n269 = Square(x=w407) -> (x^2=w408:dbl)
                n270 = Multiply(x=2.0, y=w407) -> (x*y=w406:dbl)
                n271 = Increment(x=w406) -> (x+1=w404:dbl)
                n272 = Subtract(x=w396, y=w408) -> (x-y=w403:dbl)
                n273 = Array Size(array=w401) -> (size(s)=w405:i32)
                n274 = Compound Arithmetic op=MULTIPLY(w405, invert w404, w403) -> (w397:dbl)
                n275 = Round Toward -Infinity(1:w397) -> (0:w395:dbl)
                n276 = Index Array(array=w401, index=w395) -> (element=w410:cluster{dbl, dbl})
                n277 = Decrement(x=w394) -> (x-1=w393:i32)
                n278 = Unbundle(w410) -> (w402:dbl, w399:dbl)
                n279 = Compound Arithmetic op=MULTIPLY(invert w393, w402, w396) -> (w398:dbl)
              }
            }
          }
          n280 = property on="Scanning Mode" class="Ring (strict)"("Value"=u16 1) -> ()  [unwired: 2 in, 2 out]
        }
        frame 5 {
          w418 = 6.283185307179586
          n281 = local read "Vx-max"() -> (w428:dbl)
          n282 = local read "Vy-max"() -> (w432:dbl)
          n283 = local read "Vy-max"() -> (w427:dbl)
          n284 = local read "Vx-max"() -> (w439:dbl)
          n285 = local read "Vx-min"() -> (w429:dbl)
          n286 = local read "Vy-min"() -> (w433:dbl)
          n287 = local read "Vy-min"() -> (w426:dbl)
          n288 = local read "Vx-min"() -> (w438:dbl)
          n289 = local read "Angle"() -> (w416:dbl)
          n290 = Subtract(x=w428, y=w429) -> (x-y=w430:dbl)
          n291 = Add(x=w432, y=w433) -> (x+y=w434:dbl)
          n292 = Subtract(x=w427, y=w426) -> (x-y=w425:dbl)
          n293 = Add(x=w439, y=w438) -> (x+y=w437:dbl)
          n294 = Divide(x=w430, y=2.0) -> (x/y=w422:dbl)
          n295 = Divide(x=w434, y=2.0) -> (x/y=w423:dbl)
          n296 = Divide(x=w425, y=2.0) -> (x/y=w421:dbl)
          n297 = Divide(x=w437, y=2.0) -> (x/y=w413:dbl)
          n298 = Compound Arithmetic op=MULTIPLY(w416, invert 360.0, w418) -> (w419:dbl)
          n299 = local read "points in ellipse"() -> (w420:dbl)
          n300 = Quotient & Remainder(x=w419, y=w418) -> (x-y*floor(x/y)=w415:dbl)  [unwired: 1 out]
          n301 = Negate(x=w415) -> (-x=w414:dbl)
          n302 = local write "numPixels"(w420) -> ()
          n303 = script code="t=2*pi*(1:1:N)./N;\nX=A.*cos(t).*cos(phi)-B.*sin(t).*sin(phi)+Xc\nY=A.*cos(t).*sin(phi)+B.*sin(t).*cos(phi)+Yc"("Xc"=w413, "Yc"=w423, "A"=w422, "B"=w421, "phi"=w414, "N"=w420) -> ("X"=w412:dbl[], "Y"=w411:dbl[])  [unwired: 1 in, 1 out]
        }
      }
    }
    frame #1 {
      n304 = local read "Drawing Mode"() -> (w444:u16)
      n305 = case shown="0, Default" w444 {
        tunnel: w443 -> [w448 w496]
        tunnel: w442 -> [w447 w495]
        tunnel: [w446 w496] -> w441
        tunnel: [w445 w495] -> w440
        frame 0, Default {
          n306 = flat-sequence {
            tunnel: [w456] -> w451
            tunnel: [w457] -> w452
            tunnel: w448 -> [w454]
            tunnel: w447 -> [w453]
            tunnel: [w481] -> w450
            tunnel: [w482] -> w449
            tunnel: w452 -> [w483]
            tunnel: w451 -> [w484]
            tunnel: w450 -> [w494]
            tunnel: w449 -> [w493]
            tunnel: [w494] -> w446
            tunnel: [w493] -> w445
            frame #0 {
              n307 = local read "Scanning Mode"() -> (w455:u16)
              n308 = case shown="1" w455 {
                tunnel: [w459 w463] -> w456
                tunnel: [w458 w462] -> w457
                tunnel: w454 -> [w459 w461]
                tunnel: w453 -> [w458 w460]
                frame 0, Default {
                  # "-1<x<1\n-1<y<1"
                }
                frame 1 {
                  # "0<x<1\n0<y<2pi"
                  n309 = Polar To Re/Im(2:w460, 3:w461) -> (0:w462:dbl[], 1:w463:dbl[])
                }
              }
            }
            frame #1 {
              w466 = 2.0
              n310 = local read "Vy-min"() -> (w477:dbl)
              n311 = Subtract(x="Vy-max", y=w477) -> (x-y=w479:dbl)
              n312 = Compound Arithmetic op=MULTIPLY(invert w466, w479, w483) -> (w475:dbl[])
              n313 = local read "Vx-max"() -> (w472:dbl)
              n314 = local read "Vx-min"() -> (w480:dbl)
              n315 = Subtract(x=w472, y=w480) -> (x-y=w478:dbl)
              n316 = Compound Arithmetic op=MULTIPLY(w478, w484, invert w466) -> (w476:dbl[])
              n317 = for {
                tunnel: [w492] -> w474 mode=indexing
                tunnel: [w491] -> w473 mode=indexing
                tunnel: w476 -> [w490] mode=indexing
                tunnel: w475 -> [w489] mode=indexing
                n318 = local read "Angle"() -> (w488:dbl)
                n319 = Compound Arithmetic op=MULTIPLY(6.283185307179586, w488, invert 360.0) -> (w485:dbl)
                n320 = formula code="px = xs*cos(t)+ys*sin(t);\npy = -xs*sin(t)+ys*cos(t);"("xs"=w490, "ys"=w489, "t"=w485) -> ("px"=w492:dbl, "py"=w491:dbl)
              }
              n321 = Add(x="Vy-min", y="Vy-max") -> (x+y=w467:dbl)
              n322 = local read "Vx-min"() -> (w471:dbl)
              n323 = Divide(x=w467, y=w466) -> (x/y=w468:dbl)
              n324 = Add(x=w472, y=w471) -> (x+y=w470:dbl)
              n325 = Add(x=w473, y=w468) -> (x+y=w482:dbl[])
              n326 = Divide(x=w470, y=w466) -> (x/y=w469:dbl)
              n327 = Add(x=w474, y=w469) -> (x+y=w481:dbl[])
            }
            frame #2 {
            }
          }
        }
        frame 3, 5 {
        }
      }
    }
    frame #2 {
      n328 = local read "Drawing Mode"() -> (w501:u16)
      n329 = case shown="3" w501 {
        tunnel: w500 -> [w503 w507]
        tunnel: [w503 w505] -> w499
        tunnel: [w502 w504] -> w498
        tunnel: w497 -> [w502 w506]
        frame 0, Default {
        }
        frame 3 {
          n330 = local read "points in ellipse"() -> (w508:dbl)
          n331 = Array Size(array=w507) -> (size(s)=w531:i32)
          n332 = local read "points in ellipse"() -> (w527:dbl)
          n333 = Array Size(array=w506) -> (size(s)=w523:i32)
          n334 = Decrement(x=w531) -> (x-1=w530:i32)
          n335 = Decrement(x=w523) -> (x-1=w524:i32)
          n336 = To Double Precision Float(number=w530) -> (double precision float=w529:dbl)
          n337 = local write "numPixels"(w508) -> ()
          n338 = To Double Precision Float(number=w524) -> (double precision float=w525:dbl)
          n339 = Divide(x=w529, y=w508) -> (x/y=w528:dbl)
          n340 = Divide(x=w525, y=w527) -> (x/y=w526:dbl)
          n341 = for {
            N: w508 -> [_]
            tunnel: w507 -> [w561]
            tunnel: w528 -> [w560]
            tunnel: [w559] -> w522 mode=indexing
            i -> [w557]
            n342 = Multiply(x=w560, y=w557) -> (x*y=w558:dbl)
            n343 = Interpolate 1D Array(1:w558, 2:w561) -> (0:w559:dbl)
          }
          n344 = for {
            N: w527 -> [_]
            tunnel: w506 -> [w556]
            tunnel: w526 -> [w555]
            tunnel: [w554] -> w521 mode=indexing
            i -> [w552]
            n345 = Multiply(x=w555, y=w552) -> (x*y=w553:dbl)
            n346 = Interpolate 1D Array(1:w553, 2:w556) -> (0:w554:dbl)
          }
          n347 = Rotate 1D Array(1:w522, 2:1 ("n")) -> (0:w540:dbl[])
          n348 = Rotate 1D Array(1:w521, 2:1 ("n")) -> (0:w539:dbl[])
          n349 = Subtract(x=w522, y=w540) -> (x-y=w537:dbl[])
          n350 = Subtract(x=w521, y=w539) -> (x-y=w536:dbl[])
          n351 = Square(x=w537) -> (x^2=w535:dbl[])
          n352 = Square(x=w536) -> (x^2=w534:dbl[])
          n353 = Add(x=w535, y=w534) -> (x+y=w533:dbl[])
          n354 = Square Root(x=w533) -> (sqrt(x)=w532:dbl[])
          "Y Graph 2" <- w532
          n355 = script code="a=dr2<0.00;\nwhile sum(a)>0\nb=diff(a);\nx=x(b<1);\ny=y(b<1);\nx=[x(end) x];\ny=[y(end) y];\ndr2=sqrt((diff(x)).^2+(diff(y)).^ 2)\na=dr2<0.0;\nend\nxout=x;\nyout=y;"("dr2"=w532, "x"=w522, "y"=w521) -> ("xout"=w515:dbl[], "yout"=w509:dbl[])  [unwired: 1 in, 1 out]
          n356 = local read "points in ellipse"() -> (w510:dbl)
          n357 = local read "points in ellipse"() -> (w520:dbl)
          n358 = Array Size(array=w509) -> (size(s)=w514:i32)
          n359 = Array Size(array=w515) -> (size(s)=w516:i32)
          n360 = Decrement(x=w514) -> (x-1=w513:i32)
          n361 = Decrement(x=w516) -> (x-1=w517:i32)
          n362 = To Double Precision Float(number=w513) -> (double precision float=w512:dbl)
          n363 = To Double Precision Float(number=w517) -> (double precision float=w518:dbl)
          n364 = Divide(x=w512, y=w510) -> (x/y=w511:dbl)
          n365 = Divide(x=w518, y=w520) -> (x/y=w519:dbl)
          n366 = for {
            N: w510 -> [_]
            tunnel: w509 -> [w546]
            tunnel: w511 -> [w545]
            tunnel: [w544] -> w504 mode=indexing
            i -> [w542]
            n367 = Multiply(x=w545, y=w542) -> (x*y=w543:dbl)
            n368 = Interpolate 1D Array(1:w543, 2:w546) -> (0:w544:dbl)
          }
          n369 = for {
            N: w520 -> [_]
            tunnel: w515 -> [w551]
            tunnel: w519 -> [w550]
            tunnel: [w549] -> w505 mode=indexing
            i -> [w547]
            n370 = Multiply(x=w550, y=w547) -> (x*y=w548:dbl)
            n371 = Interpolate 1D Array(1:w548, 2:w551) -> (0:w549:dbl)
          }
        }
      }
      "X-WaveArray" <- w499
      "Y-WaveArray" <- w498
    }
  }
